vi "CSM - user.lib Dir.vi"() -> (0 "<LabVIEW>":path, 1 "csm_user.lib_dir":path)   [LabVIEW 2017, in "CSM Shared.lvlib"]
uses:
  CSM Shared.lvlib
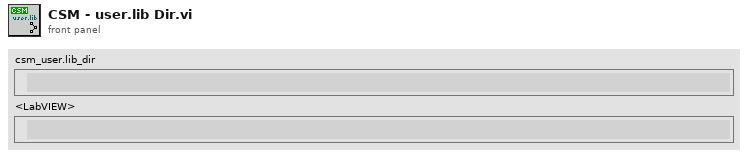
[diagram p1: front panel]
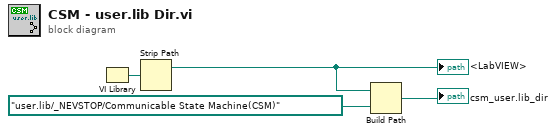
[diagram p0: block diagram]
diagram:
  n1 = VI Library() -> (path=w4:path)
  n2 = Strip Path(path=w4) -> (stripped path=w2:path)  [unwired: 1 out]
  "<LabVIEW>" <- w2
  n3 = Build Path(base path=w2, name or relative path=path "user.lib/_NEVSTOP/Communicable State Machine(CSM)" ("stripped path")) -> (appended path=→"csm_user.lib_dir":path)
